vi "Enqueue Bundled Element.vi"(6 "Priority(Low)":T1, 8 "error in":errorcluster, 10 "element":T2, 11 "QDMH in":refnum<class "QDMH.lvclass">) -> (0 "error out":errorcluster, 3 "QDMH out":refnum<class "QDMH.lvclass">)   [LabVIEW 2023, in "QDMH.lvlib" / "QDMH.lvclass"]
uses:
  QDMH.lvclass
  Custom Controls/QDMH Message.ctl
  Custom Controls/Priority.ctl
  QDMH.lvclass/QDMH.ctl
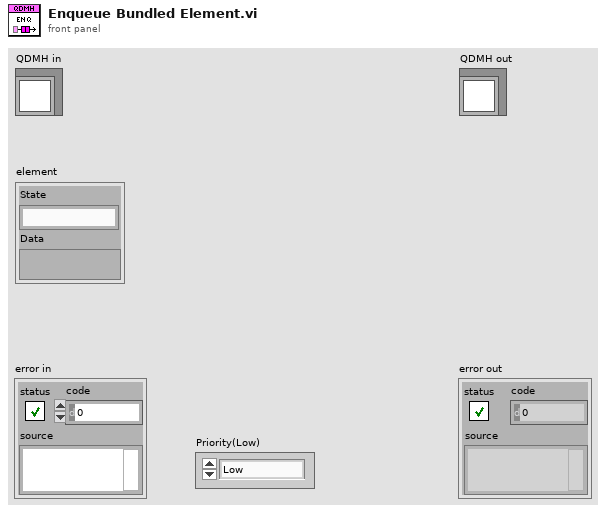
[diagram p1: front panel]
types:
  T1 = typedef "QDMH.lvlib/QDMH.lvclass/Priority.ctl" = enum16{"Low ", "High"}
  T2 = typedef "QDMH.lvlib/QDMH.lvclass/QDMH Message.ctl" = cluster{"State":string, "Data":variant}
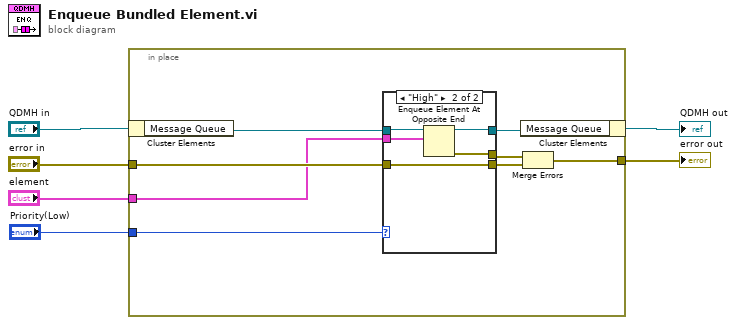
[diagram p0: block diagram]
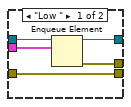
[diagram p2: hidden frame]
diagram:
  n1 = in-place {
    in-place-border: [w8] -> w5
    in-place-border: "error in" -> [w12]
    in-place-border: "element" -> [w11]
    in-place-border: "Priority(Low)" -> [w10]
    n2 = in-place-cluster #1("QDMH in") -> ("Message Queue"=w13:refnum<queue>)
    n3 = case shown="\"High\"" w10 {
      tunnel: [w19 w22] -> w14
      tunnel: w13 -> [w18 w24]
      tunnel: [w17 w21] -> w9
      tunnel: w12 -> [w15 w20]
      tunnel: w11 -> [w16 w23]
      tunnel: [w15 w20] -> w7
      frame "Low " {
        n4 = Enqueue Element(queue=w18, element=w16) -> (queue out=w19:refnum<queue>, error out=w17:errorcluster)  [unwired: 2 in, 1 out]
      }
      frame "High" {
        n5 = Enqueue Element At Opposite End(queue=w24, element=w23) -> (queue out=w22:refnum<queue>, error out=w21:errorcluster)  [unwired: 2 in, 1 out]
      }
    }
    n6 = in-place-cluster #1("Message Queue"=w14) -> (→"QDMH out":refnum<class "QDMH.lvclass">)
    n7 = Merge Errors(w9, w7) -> (w8:errorcluster)
  }
  "error out" <- w5
